vi "Write MFC_.vi"(8 "error in (no error)":errorcluster, 10 "MFC?":bool, 11 "Purge Switch MSG in":refnum<class "Purge Switch MSG.lvclass">) -> (0 "error out":errorcluster, 3 "Purge Switch MSG out":refnum<class "Purge Switch MSG.lvclass">)   [LabVIEW 2014]
uses:
  Purge Switch MSG.lvclass
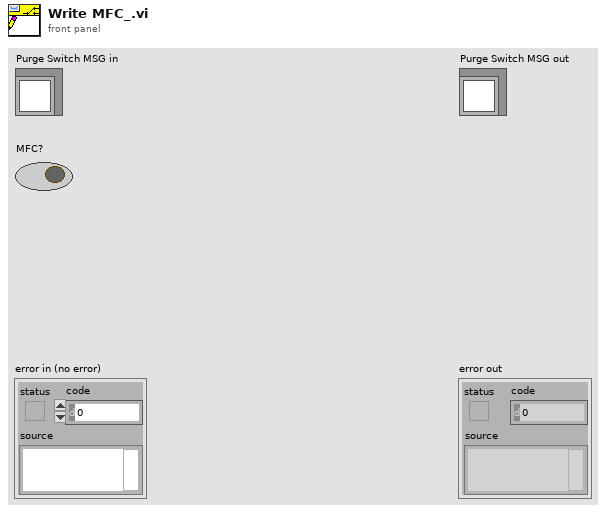
[diagram p1: front panel]
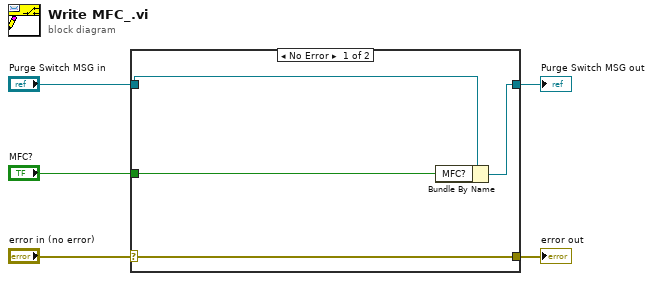
[diagram p0: block diagram]
diagram:
  n1 = case shown="No Error" "error in (no error)" {
    selector: "error in (no error)" -> [w9 w10]
    tunnel: [w9 w10] -> w4
    tunnel: [w7 w11] -> w2
    tunnel: "Purge Switch MSG in" -> [w8 w11]
    tunnel: "MFC?" -> [w6 _]
    frame No Error {
      n2 = Bundle By Name(cluster=w8, "MFC?"=w6) -> (w7:refnum<class "Purge Switch MSG.lvclass">)
    }
    frame Error {
    }
  }
  "error out" <- w4
  "Purge Switch MSG out" <- w2
